vi "Energy to Elevation_cubic_subVI.vi"(11 "Puck Energy Requirement (mJ)":dbl) -> ()   [LabVIEW 2017]
uses:
  <vilib>/Analysis/polynomials.llb/Polynomial Roots (DBL).vi
  <vilib>/Analysis/NI_AALPro.lvlib
panel:
  out "Output Velocity":dbl
  out "Pull-back angle 3":dbl
  out "Pull-back angle 2":dbl
  out "Pull-back angle":dbl
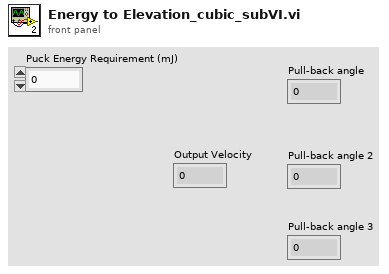
[diagram p1: front panel]
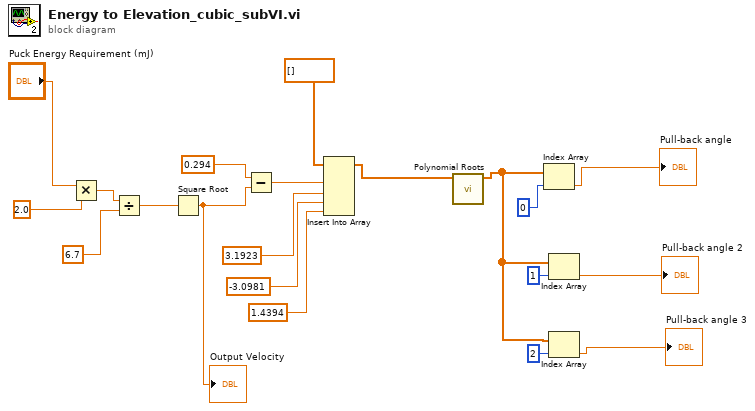
[diagram p0: block diagram]
diagram:
  n1 = Multiply(x="Puck Energy Requirement (mJ)", y=2.0) -> (x*y=w18:dbl)
  n2 = Divide(x=w18, y=6.7) -> (x/y=w20:dbl)
  n3 = Square Root(x=w20) -> (sqrt(x)=w1:dbl)
  "Output Velocity" <- w1
  n4 = Subtract(x=0.294 ("new element/subarray"), y=w1) -> (x-y=w9:dbl)
  n5 = Insert Into Array(array=dbl[] [], new element #1=w9, new element #2=3.1923 ("new element/subarray"), new element #3=-3.0981 ("new element/subarray"), new element #4=1.4394 ("new element/subarray")) -> (w11:dbl[])  [unwired: 1 in]
  n6 = call-poly <vilib>:"Polynomial Roots.vi"("P(x)"=w11) -> ("Roots"=w3:cdb[])  [unwired: 9 in, 1 out]
  n7 = Index Array(array=w3, index=0) -> (element=→"Pull-back angle":cdb)
  n8 = Index Array(array=w3, index=1) -> (element=→"Pull-back angle 2":cdb)
  n9 = Index Array(array=w3, index=2) -> (element=→"Pull-back angle 3":cdb)
